vi "Connect COM Port (SubVI).vi"(8 "error in (no error)":errorcluster) -> (0 "error out":errorcluster, 2 "NoCOM PORT":bool caption="OK", 3 "VISA Refnum out":refnum<visa-resource-name>)   [LabVIEW 2017]
uses:
  <vilib>/Instr/_visa.llb/VISA Configure Serial Port (Instr).vi
panel:
  out "COM only list":string[](array[string])
  out "Original list":string[](array[string])
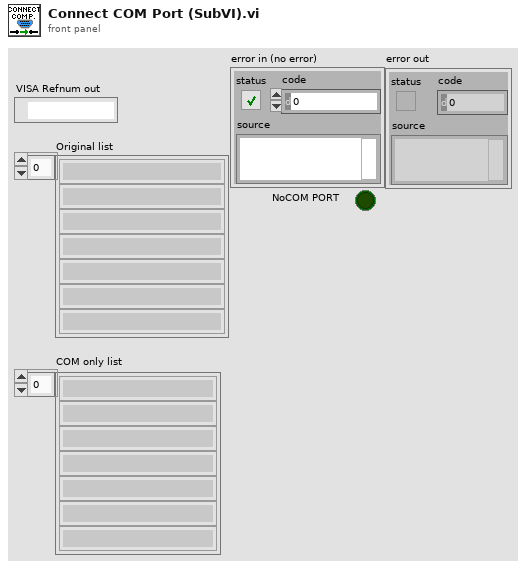
[diagram p1: front panel]
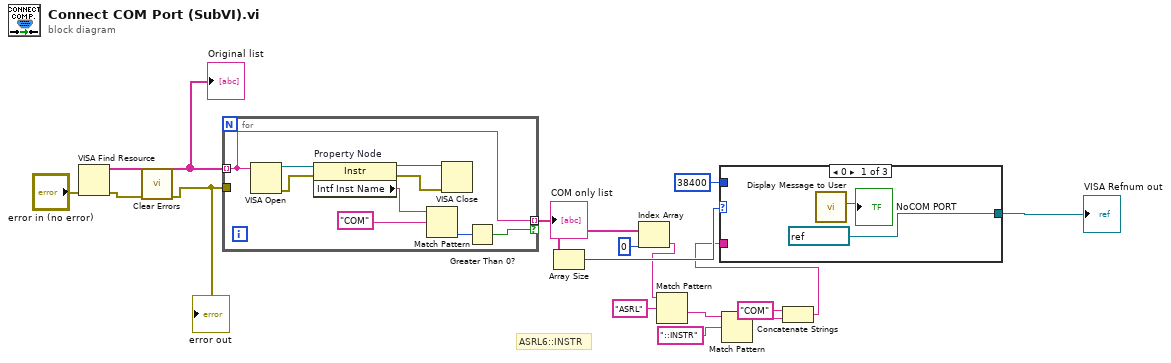
[diagram p0: block diagram]
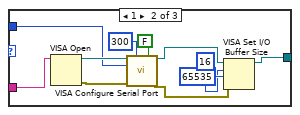
[diagram p2: hidden frame]
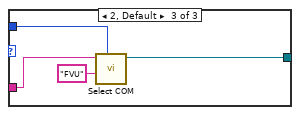
[diagram p3: hidden frame]
diagram:
  # "ASRL6::INSTR"
  n1 = VISA Find Resource(8:"error in (no error)") -> (0:w10:errorcluster, 3:w9:string[])  [unwired: 2 in, 1 out]
  "Original list" <- w9
  n2 = call <vilib>:"Clear Errors.vi"("error in (no error)"=w10) -> ("error out"=w11:errorcluster)  [unwired: 5 in, 1 out]
  "error out" <- w11
  n3 = for {
    tunnel: w9 -> [w19] mode=indexing
    tunnel: [w19] -> w14 mode=indexing if=w17
    tunnel: w11 -> [_]
    n4 = VISA Open(VISA resource name=w19) -> (VISA resource name=w25:refnum<visa-resource-name>, error out=w24:errorcluster)  [unwired: 4 in]
    n5 = property on="Property Node" class="Instr"(reference=w25, error in=w24) -> (reference out=w23:refnum<visa-resource-name>, error out=w22:errorcluster, "Intf Inst Name"=w21:string)
    n6 = Match Pattern(string=w21, regular expression="COM") -> (offset past match=w18:i32)  [unwired: 1 in, 3 out]
    n7 = VISA Close(VISA resource name=w23, error in (no error)=w22) -> ()  [unwired: 1 out]
    n8 = Greater Than 0?(x=w18) -> (x > 0?=w17:bool)
  }
  "COM only list" <- w14
  n9 = Array Size(array=w14) -> (size(s)=w12:i32)
  n10 = Index Array(array=w14, index=0) -> (element=w7:string)
  n11 = Match Pattern(string=w7, regular expression="ASRL") -> (after substring=w5:string)  [unwired: 1 in, 3 out]
  n12 = Match Pattern(string=w5, regular expression="::INSTR") -> (before substring=w3:string)  [unwired: 1 in, 3 out]
  n13 = Concatenate Strings("COM" ("string"), w3) -> (w1:string)
  n14 = case shown="0" w12 {
    tunnel: u32 38400 ("baud rate") -> [_ w35 w42]
    tunnel: [refnum<visa-resource-name> "COMx" ("VISA resource name out") w28 w40] -> w16
    tunnel: w1 -> [_ w33 w39]
    frame 0 {
      n15 = call "Display Message to User"() -> ("OK"=→"NoCOM PORT":bool)  [unwired: 10 in, 1 out]
    }
    frame 1 {
      n16 = VISA Open(VISA resource name=w33) -> (VISA resource name=w36:refnum<visa-resource-name>, error out=w34:errorcluster)  [unwired: 4 in]
      n17 = call-poly "VISA Configure Serial Port"("VISA resource name"=w36, "timeout (10sec)"=u32 300, "Enable Termination\nChar (T)"=FALSE ("Enable Termination\nChar (T)"), "baud rate (9600)"=w35, "error in (no error)"=w34) -> ("VISA resource name out"=w31:refnum<visa-resource-name>, "error out"=w29:errorcluster)  [unwired: 9 in]
      n18 = VISA Set I/O Buffer Size(VISA resource name=w31, mask (16)=u16 16, size (4096)=u32 65535, error in (no error)=w29) -> (VISA resource name out=w28:refnum<visa-resource-name>)  [unwired: 1 out]
    }
    frame 2, Default {
      n19 = call "Select COM.vi"("baud rate"=w42, "Port Name"="FVU", "VISA resource name 2"=w39) -> ("VISA resource name out"=w40:refnum<visa-resource-name>)  [unwired: 6 in, 2 out]
    }
  }
  "VISA Refnum out" <- w16
